vi "Delacor_lib_QMH_Enqueue Message (poly).vi"   [LabVIEW 2024, in "RQMHMessageQueue.lvclass"]
doc: "For a regular message, enqueue the message. For a priority message, enqueue it at the front of the queue.\n____\nDQMH Framework: Palette 7.1.0.1503\nCopyright (c) 2025, DQMH Consortium"
uses:
  RQMHMessageQueue.lvclass
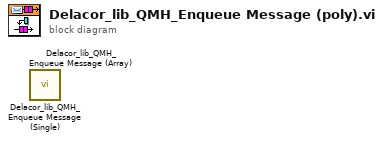
[diagram p0: block diagram]
diagram:
  n1 = call "Delacor_lib_QMH_Enqueue Message (Single).vi"() -> ()  [unwired: 10 in, 2 out]
  n2 = call "Delacor_lib_QMH_Enqueue Message (Array).vi"() -> ()  [unwired: 10 in, 2 out]
